vi "Actor Core.vi"(8 "error in":errorcluster, 11 "IO Device in":refnum<class "IO Device.lvclass">) -> (0 "error out":errorcluster, 3 "Actor out":refnum<class "Actor.lvclass">)   [LabVIEW 2015, in "IO Device.lvlib" / "IO Device.lvclass"]
doc: "(<B>Filename</B>: Actor Framework.lvlib:Actor.lvclass:Actor Core.vi)\n\nReceives messages to the actor, reacts to them, and initiates any error handling that may shut the actor down.\n\nDescendant classes may override this VI to append parallel tasks for the actor to complete while it handles messages. Overrides use the Call Parent Method node."
uses:
  IO Device.lvclass
  <vilib>/ActorFramework/Actor/Actor.lvclass
  <vilib>/MGI/Monitored Actor/Monitored Actor/Monitored Actor/Monitored Actor.lvclass
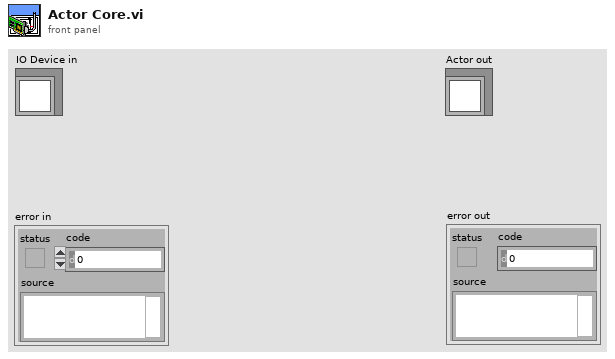
[diagram p1: front panel]
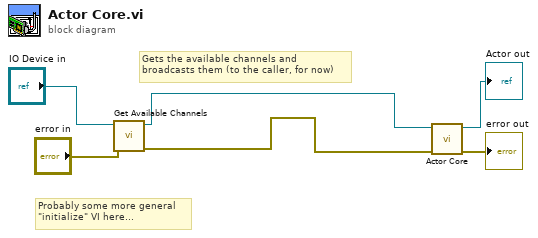
[diagram p0: block diagram]
diagram:
  # "Gets the available channels and \nbroadcasts them (to the caller, for now)"
  # "Probably some more general\n\"initialize\" VI here..."
  n1 = call-dynamic "Get Available Channels.vi"("error in (no error)"="error in", "IO Device in"="IO Device in") -> ("error out"=w1:errorcluster, "IO Device out"=w2:refnum<class "IO Device.lvclass">)  [unwired: 8 in]
  n2 = call-parent "Actor Core.vi"("error in"=w1, "Actor in"=w2) -> ("error out"=→"error out":errorcluster, "Actor out"=→"Actor out":refnum<class "Actor.lvclass">)  [unwired: 8 in]
